vi "handler_home.vi"(8 "error in (no error)":errorcluster, 10 "Server Variables":T1 {"Energy Levels"."E1" format="%_6g"; "Phases"."ExtTriggerDelay" format="%.3g"}, 11 "HTTP Request in":T7) -> (0 "error out":errorcluster, 2 "Server Variables":T1 {"Energy Levels"."E1" format="%_6g"; "Phases"."ExtTriggerDelay" format="%.3g"}, 3 "HTTP Request out":T7)   [LabVIEW 2011]
uses:
  http_request_response.ctl
  http_request.ctl
  http_field.ctl
  http_response.ctl
  template_field.ctl
  template_field_type.ctl
  Server Variables.ctl
  Phase Parameters.ctl
  Phase Mode.ctl
  Energy Level_.ctl
  Measurement Parameters.ctl
  Results.ctl
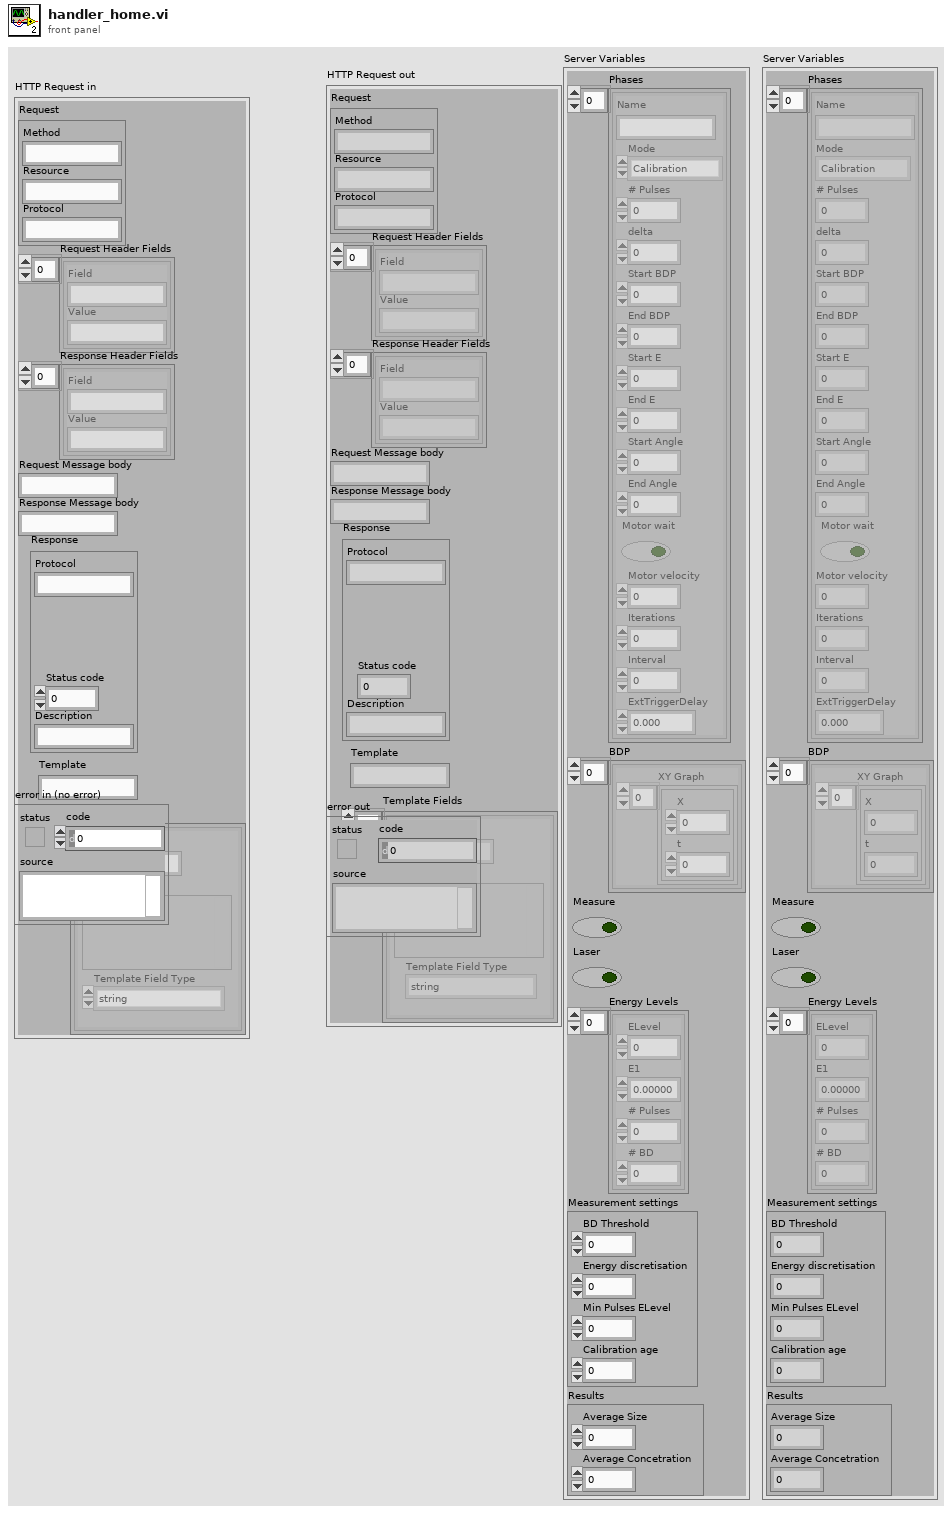
[diagram p1: front panel]
types:
  T1 = typedef "Server Variables.ctl" = cluster{"Phases":T2[], "BDP":cluster{"XY Graph":cluster{"X":dbl, "t":dbl}[]}[], "Measure":bool, "Laser":bool, "Energy Levels":T4[], "Measurement settings":T5, "Results":T6}
  T2 = typedef "Phase Parameters.ctl" = cluster{"Name":string, "Mode":T3, "# Pulses":u32, "delta":dbl, "Start BDP":dbl, "End BDP":dbl, "Start E":dbl, "End E":dbl, "Start Angle":dbl, "End Angle":dbl, "Motor wait":bool, "Motor velocity":dbl, "Iterations":dbl, "Interval":dbl, "ExtTriggerDelay":dbl}
  T3 = typedef "Phase Mode.ctl" = enum16{"Calibration", "Linear", "BDP-Fit", "Raw"}
  T4 = typedef "Energy Level_.ctl" = cluster{"ELevel":dbl, "E1":dbl, "# Pulses":i32, "# BD":i32}
  T5 = typedef "Measurement Parameters.ctl" = cluster{"BD Threshold":dbl, "Energy discretisation":i32, "Min Pulses ELevel":i32, "Calibration age":i32}
  T6 = typedef "Results.ctl" = cluster{"Average Size":dbl, "Average Concetration":dbl}
  T7 = typedef "http_request_response.ctl" = cluster{"Request":T8, "Request Header Fields":T9[], "Response Header Fields":T9[], "Request Message body":string, "Response Message body":string, "Response":T10, "Template":string, "Template Fields":T11[]}
  T8 = typedef "http_request.ctl" = cluster{"Method":string, "Resource":string, "Protocol":string}
  T9 = typedef "http_field.ctl" = cluster{"Field":string, "Value":string}
  T10 = typedef "http_response.ctl" = cluster{"Protocol":string, "Status code":dbl, "Description":string}
  T11 = typedef "template_field.ctl" = cluster{"Name":string, "Template Field Type":T12, "data":variant}
  T12 = typedef "template_field_type.ctl" = enum16{"string", "string array", "number", "number array", "cluster", "cluster array"}
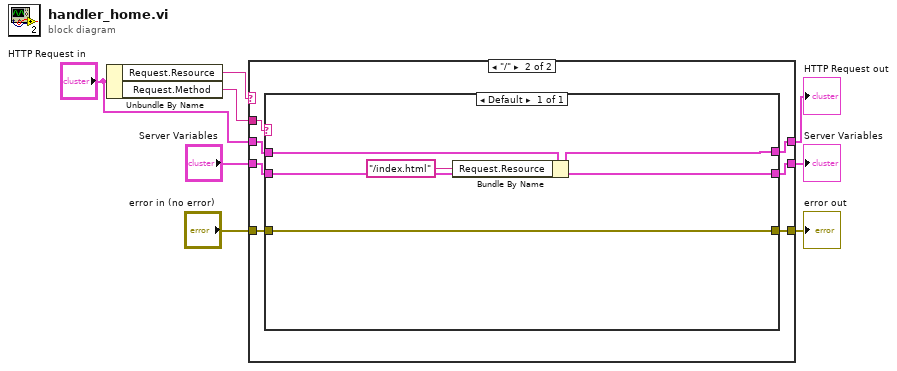
[diagram p0: block diagram]
diagram:
  n1 = Unbundle By Name("HTTP Request in") -> ("Request.Resource"=w8:string, "Request.Method"=w7:string)
  n2 = case shown="\"/\"" w8 {
    tunnel: w7 -> [_ w18]
    tunnel: "HTTP Request in" -> [w11 w17]
    tunnel: [w11 w16] -> w5
    tunnel: "error in (no error)" -> [w10 w15]
    tunnel: [w10 w14] -> w3
    tunnel: "Server Variables" -> [w9 w13]
    tunnel: [w9 w12] -> w1
    frame Default {
    }
    frame "/" {
      n3 = case shown="Default" w18 {
        tunnel: w17 -> [w23]
        tunnel: [w20] -> w16
        tunnel: w15 -> [w22]
        tunnel: [w22] -> w14
        tunnel: w13 -> [w21]
        tunnel: [w21] -> w12
        frame Default {
          n4 = Bundle By Name(cluster=w23, "Request.Resource"="/index.html") -> (w20:T7)
        }
      }
    }
  }
  "HTTP Request out" <- w5
  "error out" <- w3
  "Server Variables" <- w1
